vi "Read.vi"(8 "error in (no error)":errorcluster, 11 "NI Vision Camera in":refnum<class "NI Vision Camera.lvclass">) -> (0 "error out":errorcluster, 1 "timed out?":bool=TRUE, 2 "Data":refnum<class "AbstractData.lvclass">, 3 "NI Vision Camera out":refnum<class "NI Vision Camera.lvclass">)   [LabVIEW 2014, in "NI Vision Camera.lvclass"]
uses:
  NI Vision Camera.lvclass
  Framework/Model/Data/AbstractData/AbstractData.lvclass
  Framework/Model/Data/Data2D/Data2D.lvclass
  NI Vision Camera.lvclass/NI Vision Camera.ctl
  Framework/Interfaces/Observable Actor/Observable Actor.lvclass
  <vilib>/vision/driver/NI_Vision_Acquisition_Software.lvlib
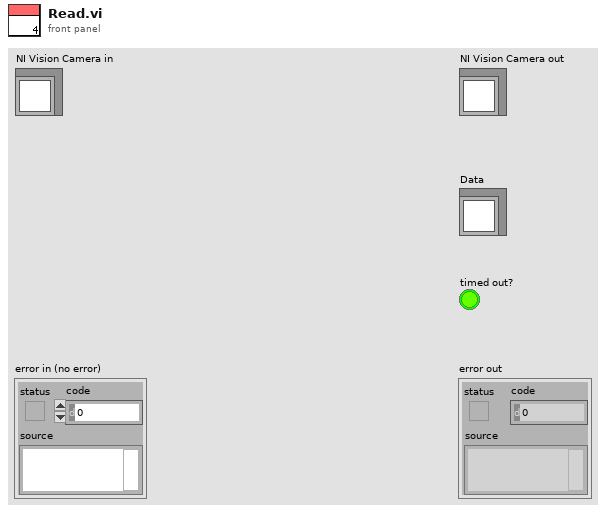
[diagram p1: front panel]
types:
  T1 = typedef "Image Type" = u32
  T2 = typedef "IMAQdx.ctl" = refnum<k21>
  T3 = typedef "IMAQ Image.ctl" = refnum<image>
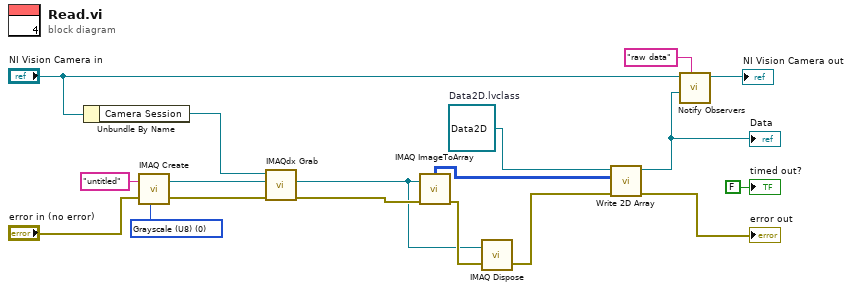
[diagram p0: block diagram]
diagram:
  w7 = T1 0 items=["Grayscale (U8)", "Grayscale (I16)", "Grayscale (SGL)", "Complex (CSG)", "RGB (U32)", "HSL (U32)", "RGB (U64)", "Grayscale (U16)"] ("Image Type")
  w18 = refnum<class "Data2D.lvclass"> refnum  # Data2D.lvclass
  n1 = Unbundle By Name("NI Vision Camera in") -> ("Camera Session"=w12:T2)
  n2 = call "IMAQ Create"("Image Name"="untitled", "Image Type"=w7, "error in (no error)"="error in (no error)") -> ("New Image"=w10:T3, "error out"=w8:errorcluster)  [unwired: 2 in]
  n3 = call <vilib>:"IMAQdx Grab.vi"("error in"=w8, "Image In"=w10, "Session In"=w12) -> ("error out"=w6:errorcluster, "Image Out"=w4:T3)  [unwired: 5 in, 2 out]
  n4 = call "IMAQ ImageToArray"("error in (no error)"=w6, "Image"=w4) -> ("error out"=w5:errorcluster, "Image Pixels (U8)"=w3:u8[][])  [unwired: 2 in, 3 out]
  n5 = call "IMAQ Dispose"("Image"=w4, "error in (no error)"=w5) -> ("error out"=w2:errorcluster)  [unwired: 4 in]
  n6 = call "Write 2D Array.vi"("error in (no error)"=w2, "2D Array"=w3, "Data2D in"=w18) -> ("error out"=→"error out":errorcluster, "Data2D out"=w14:refnum<class "Data2D.lvclass">)  [unwired: 7 in]
  "Data" <- w14
  n7 = call "Notify Observers.vi"("name"="raw data", "value"=w14, "Observable Actor in"="NI Vision Camera in") -> ("Observable Actor out"=→"NI Vision Camera out":refnum<class "NI Vision Camera.lvclass">)  [unwired: 7 in, 1 out]
  "timed out?" <- FALSE ("timed out?")
